vi "simulate_keyboard.vi"(7 "error in (no error)":errorcluster, 9 "Direction":enum16{"Key Down", "Key Up"}(ring), 10 "Virtual Key":u8(ring)=165) -> (0 "error out":errorcluster)   [LabVIEW 2015, in "LVJSON.lvlib" / "Shared.lvlib"]
doc: "This VI simulates Keyboard events by making calls into the keyb_event function of the Windows User32.dll\n\nInstructions:\n1) Run the program\n2) Press the keys in the order you would like to simulate them\n Example 1: With several applications open, press Alt, Tab, Tab, Tab, Alt\n Example 2: Alt, F, Alt, O, A, B, C\n3) Press the Execute button to watch the code simulate the keyboard events"
uses:
  Shared.lvlib
  user32.dll
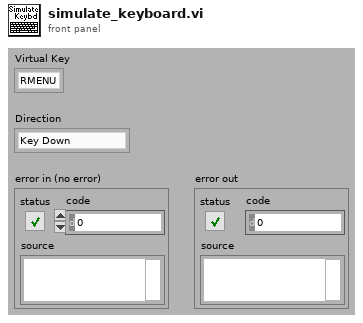
[diagram p1: front panel]
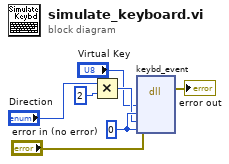
[diagram p0: block diagram]
diagram:
  w5 = u32 0 ("dwFlags")
  n1 = Multiply(x="Direction", y=2) -> (x*y=w4:i32)
  n2 = dll-call lib="user32.dll" fn="keybd_event"(error in="error in (no error)", "bVk"="Virtual Key", "bScan"=w5, "dwFlags"=w4, "dwExtraInfo"=w5) -> (error out=→"error out":errorcluster)  [unwired: 7 in, 1 out]
